vi "Configure Serial Bus (MANC - Decode).vi"(0 "VISA resource name":refnum<visa-resource-name>, 1 "Word Size (8)":i32=8, 2 "Display Type (1: Word)":i32(ring)=1 items=["Bit", "Word"], 5 "Serial Bus Name (1: Serial Bus 1)":i32(ring)=1 items=["Serial Bus 1"=1, "Serial Bus 2"=2], 7 "Decode Base (0: Hexadecimal)":i32(ring) items=["Hexadecimal", "Unsigned Decimal", "ASCII", "Binary"], 9 "Bit Order (0: Most Significant Bit First )":i32(ring) items=["Most Significant Bit First ", "Least Significant Bit First"], 11 "error in (no error)":errorcluster, 12 "Data Size (1)":i32=1, 13 "Header Size (0)":i32, 14 "Trailer Size (0)":i32) -> (4 "VISA resource name out":refnum<visa-resource-name>, 15 "error out":errorcluster)   [LabVIEW 2015, in "Agilent 2000 3000 X-Series.lvlib"]
doc: "Configures the display setting of Manchester bus.\n\n<b>Note:</b>\nThis VI is only applicable for 3000T, 4000, 6000 X-Series."
uses:
  Agilent 2000 3000 X-Series.lvlib
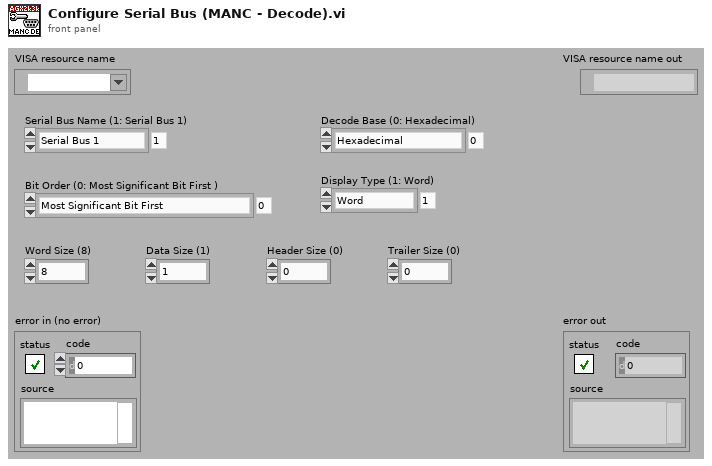
[diagram p1: front panel]
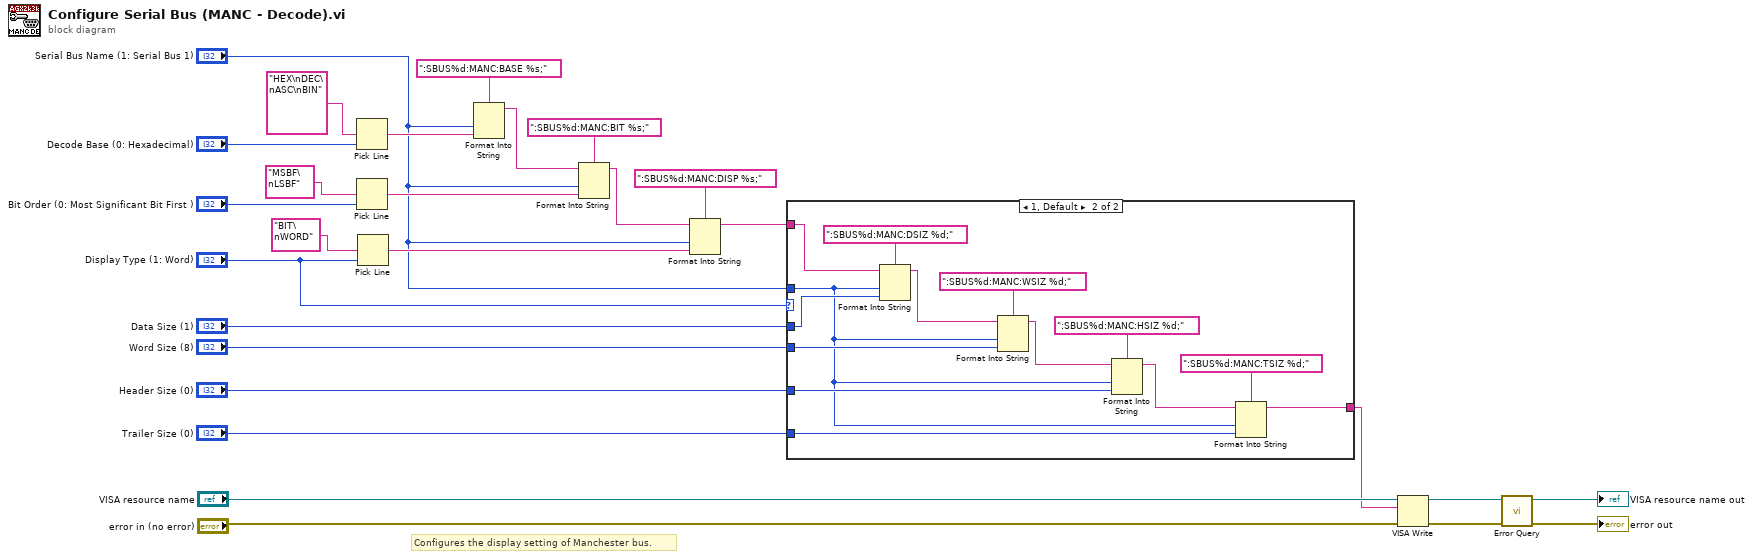
[diagram p0: block diagram]
diagram:
  # "Configures the display setting of Manchester bus."
  n1 = Pick Line(multi-line string="HEX\nDEC\nASC\nBIN", line index="Decode Base (0: Hexadecimal)") -> (output string=w20:string)  [unwired: 1 in]
  n2 = Pick Line(multi-line string="MSBF\nLSBF", line index="Bit Order (0: Most Significant Bit First )") -> (output string=w24:string)  [unwired: 1 in]
  n3 = Pick Line(multi-line string="BIT\nWORD", line index="Display Type (1: Word)") -> (output string=w10:string)  [unwired: 1 in]
  n4 = Format Into String(format string=":SBUS%d:MANC:BASE %s;", "Serial Bus Name (1: Serial Bus 1)", w20) -> (resulting string=w13:string)  [unwired: 2 in, 1 out]
  n5 = Format Into String(format string=":SBUS%d:MANC:BIT %s;", initial string=w13, "Serial Bus Name (1: Serial Bus 1)", w24) -> (resulting string=w9:string)  [unwired: 1 in, 1 out]
  n6 = Format Into String(format string=":SBUS%d:MANC:DISP %s;", initial string=w9, "Serial Bus Name (1: Serial Bus 1)", w10) -> (resulting string=w6:string)  [unwired: 1 in, 1 out]
  n7 = case shown="1, Default" "Display Type (1: Word)" {
    tunnel: "Serial Bus Name (1: Serial Bus 1)" -> [_ w32]
    tunnel: w6 -> [w28 w38]
    tunnel: "Data Size (1)" -> [_ w37]
    tunnel: "Word Size (8)" -> [_ w35]
    tunnel: "Header Size (0)" -> [_ w33]
    tunnel: "Trailer Size (0)" -> [_ w31]
    tunnel: [w28 w29] -> w1
    frame 0 {
    }
    frame 1, Default {
      n8 = Format Into String(format string=":SBUS%d:MANC:DSIZ %d;", initial string=w38, w32, w37) -> (resulting string=w36:string)  [unwired: 1 in, 1 out]
      n9 = Format Into String(format string=":SBUS%d:MANC:WSIZ %d;", initial string=w36, w32, w35) -> (resulting string=w34:string)  [unwired: 1 in, 1 out]
      n10 = Format Into String(format string=":SBUS%d:MANC:HSIZ %d;", initial string=w34, w32, w33) -> (resulting string=w30:string)  [unwired: 1 in, 1 out]
      n11 = Format Into String(format string=":SBUS%d:MANC:TSIZ %d;", initial string=w30, w32, w31) -> (resulting string=w29:string)  [unwired: 1 in, 1 out]
    }
  }
  n12 = VISA Write(VISA resource name="VISA resource name", write buffer=w1, error in (no error)="error in (no error)") -> (VISA resource name out=w17:refnum<visa-resource-name>, error out=w16:errorcluster)  [unwired: 1 out]
  n13 = call "Error Query.vi"("error in (no error)"=w16, "VISA resource name"=w17) -> ("error out"=→"error out":errorcluster, "VISA resource name out"=→"VISA resource name out":refnum<visa-resource-name>)  [unwired: 6 in, 2 out]
